vi "Enable Multiple High Voltage Channels.vi"(8 "error in (no error)":errorcluster, 10 "High Voltage Channels":i32[](array[numeric]), 11 "VISA resource name":refnum<visa-resource-name>) -> (0 "error out":errorcluster, 3 "VISA resource name out":refnum<visa-resource-name>)   [LabVIEW 2014, in "Associated Research SC6540.lvlib"]
doc: "Connect the specified channels to high voltage port. The other channels will not be changed."
uses:
  <instrlib>/Associated Research SC6540/Associated Research SC6540.lvlib
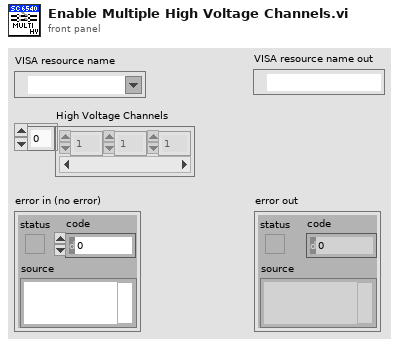
[diagram p1: front panel]
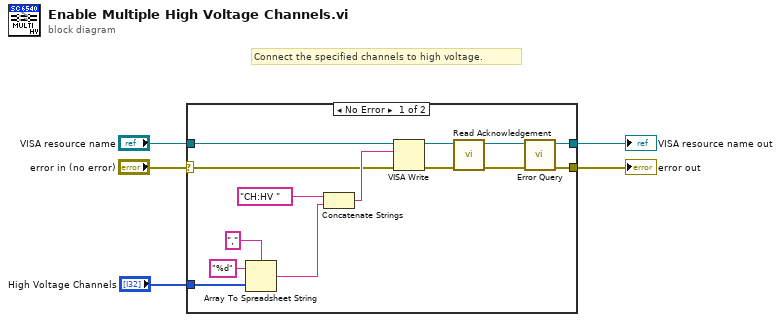
[diagram p0: block diagram]
diagram:
  # "Connect the specified channels to high voltage."
  n1 = case shown="No Error" "error in (no error)" {
    selector: "error in (no error)" -> [w6 w21]
    tunnel: "VISA resource name" -> [w19 w20]
    tunnel: [w14 w20] -> w4
    tunnel: [w13 w21] -> w3
    tunnel: "High Voltage Channels" -> [w12 _]
    frame No Error {
      n2 = Array To Spreadsheet String(delimiter (Tab)=",", array=w12, 3:"%d" ("format string")) -> (spreadsheet string=w9:string)
      n3 = Concatenate Strings("CH:HV " ("command"), w9) -> (w7:string)
      n4 = VISA Write(VISA resource name=w19, write buffer=w7, error in (no error)=w6) -> (VISA resource name out=w18:refnum<visa-resource-name>, error out=w17:errorcluster)  [unwired: 1 out]
      n5 = call <instrlib>:"Read Acknowledgement.vi"("error in (no error)"=w17, "VISA resource name"=w18) -> ("error out"=w15:errorcluster, "VISA resource name out"=w16:refnum<visa-resource-name>)  [unwired: 8 in]
      n6 = call <instrlib>:"Error Query.vi"("error in (no error)"=w15, "VISA resource name"=w16) -> ("error out"=w13:errorcluster, "VISA resource name out"=w14:refnum<visa-resource-name>)  [unwired: 6 in, 2 out]
    }
    frame Error {
    }
  }
  "VISA resource name out" <- w4
  "error out" <- w3
